vi "ColorRamp_viaPropNodes 2012 NIVerified.vi"() -> ()   [LabVIEW 2019]
doc: "This example shows how to programmatically change the colors of the markers using property nodes."
panel:
  in  "Past Lower Limit Color":u32(colorbox)=16448250
  in  "Past Upper Limit Color":u32(colorbox)
  in  "Knob":dbl(knob) scale=-1.0..101.0
  in  "stop":bool
  out "Color Ramp":dbl(ramp)
  out "Maker Values OUTPUT":cluster{dbl, u32}[](array[cluster])
  in  "Maker Values INPUT":cluster{dbl, u32}[](array[cluster])=[{0.0, 6618880}, {50.0, 16318208}, {100.0, 16711680}]
  # "Overview: This example shows how to programmatically change the colors of the markers using property nodes.\nInstruction: \n1) Run the VI.\n2) Move the Knob Control to see how the Color Ramp Responds.\n3) You can change any of the colors, such as marker colors or the extreme range colors.\nAll of this can be done via the front panel, also. To change the colors, the Marker Spacing needs to be set to Arbitrary."
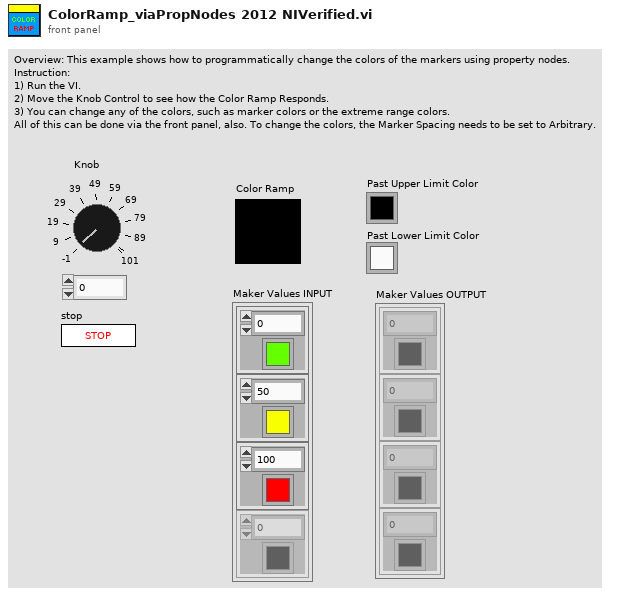
[diagram p1: front panel]
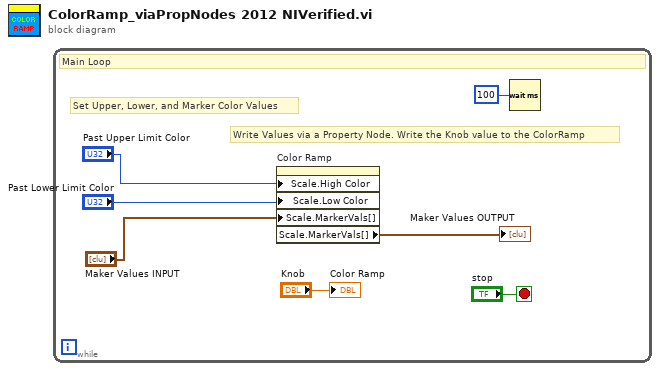
[diagram p0: block diagram]
diagram:
  n1 = while {
    stop <- "stop" stop-if-true
    # "Write Values via a Property Node. Write the Knob value to the ColorRamp"
    # "Set Upper, Lower, and Marker Color Values"
    # "Main Loop"
    n2 = property on="Color Ramp" class="ColRmp (strict)"("Scale.High Color"="Past Upper Limit Color", "Scale.Low Color"="Past Lower Limit Color", "Scale.MarkerVals[]"="Maker Values INPUT") -> ("Scale.MarkerVals[]"=→"Maker Values OUTPUT":cluster{dbl, u32}[])  [unwired: 2 in, 2 out]
    n3 = Wait (ms)(milliseconds to wait=u32 100) -> ()  [unwired: 1 out]
    "Color Ramp" <- "Knob"
  }
